vi "output_data.vi"(8 "dimension size":i32=16, 9 "O/p Name":string[](array[string]), 10 "Digital Output_in":T1(array[cluster])) -> (1 "No of Row":i32=16, 2 "Digital Output":T1(array[cluster]))   [LabVIEW 2015]
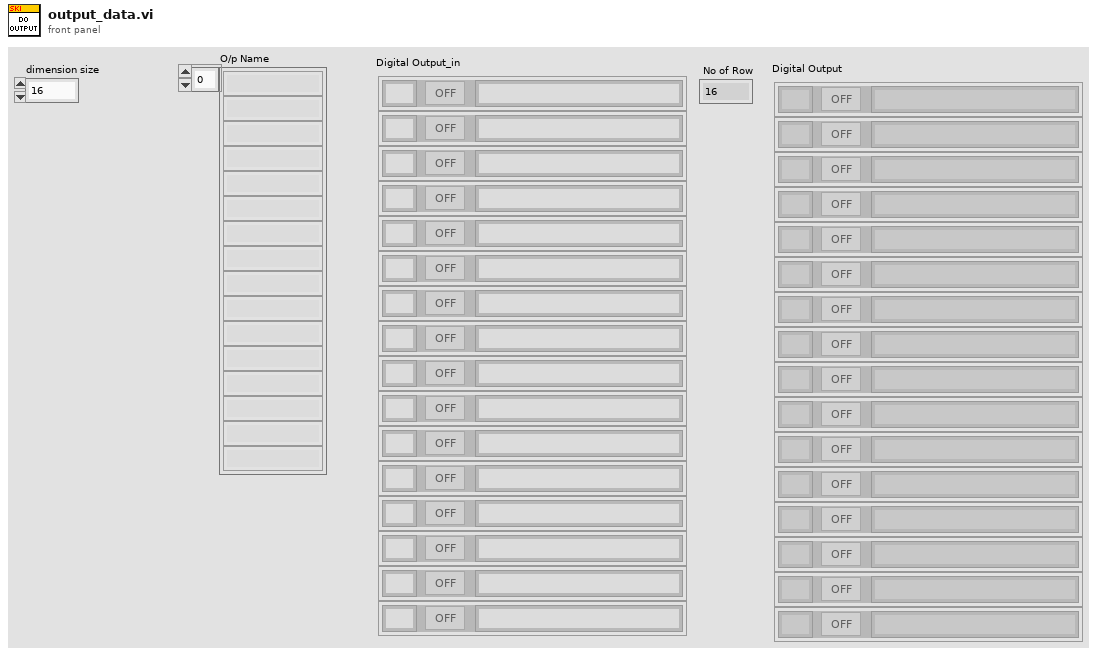
[diagram p1: front panel]
types:
  T1 = cluster{"Name":string, "Output":bool, "S.N0":string}[]
  T2 = cluster{"Name":string, "Output":bool, "S.N0":string}
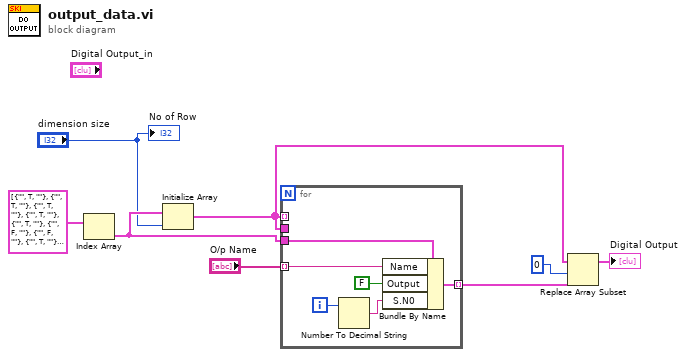
[diagram p0: block diagram]
diagram:
  n1 = Index Array(array=T1 [{"Name"="", "Output"=TRUE, "S.N0"=""}, {"Name"="", "Output"=TRUE, "S.N0"=""}, {"Name"="", "Output"=TRUE, "S.N0"=""}, {"Name"="", "Output"=TRUE, "S.N0"=""}, {"Name"="", "Output"=TRUE, "S.N0"=""}, {"Name"="", "Output"=FALSE, "S.N0"=""}, {"Name"="", "Output"=FALSE, "S.N0"=""}, {"Name"="", "Output"=TRUE, "S.N0"=""}, {"Name"="", "Output"=FALSE, "S.N0"=""}, {"Name"="", "Output"=TRUE, "S.N0"=""}, {"Name"="", "Output"=TRUE, "S.N0"=""}, {"Name"="", "Output"=TRUE, "S.N0"=""}, {"Name"="", "Output"=FALSE, "S.N0"=""}, {"Name"="", "Output"=FALSE, "S.N0"=""}, {"Name"="", "Output"=TRUE, "S.N0"=""}, {"Name"="", "Output"=TRUE, "S.N0"=""}, {"Name"="", "Output"=TRUE, "S.N0"=""}] ("Array 4")) -> (element=w7:T2)  [unwired: 1 in]
  n2 = Initialize Array(w7, "dimension size") -> (w6:T1)
  n3 = for {
    tunnel: w6 -> [_] mode=indexing
    tunnel: w6 -> [_]
    tunnel: w7 -> [w14]
    tunnel: [w10] -> w5 mode=indexing
    tunnel: "O/p Name" -> [w9] mode=indexing
    i -> [w13]
    n4 = Number To Decimal String(number=w13) -> (decimal integer string=w12:string)  [unwired: 1 in]
    n5 = Bundle By Name(cluster=w14, "Name"=w9, "Output"=FALSE, "S.N0"=w12) -> (w10:T2)
  }
  n6 = Replace Array Subset(array=w6, new element=w5, index=0) -> (→"Digital Output":T1)
  "No of Row" <- "dimension size"
